vi "GetCreditTransactions.vi"(8 "error in (no error)":errorcluster, 9 "Month":T1, 10 "YYYY":i32, 11 "Account History in":refnum<class "Account History.lvclass">) -> (0 "error out":errorcluster, 2 "Credit Transactions.lvclass":refnum<class "Credit Transactions.lvclass">, 3 "Account History out":refnum<class "Account History.lvclass">)   [LabVIEW 2018, in "Account History.lvclass"]
uses:
  Account History.lvclass
  Credit Statement/Credit Transactions.lvclass
  C:/GitRepos/Filthy-Lucre-Budgetizer/source/support/classes/Statement/TransactionList.lvclass
  Month.ctl
  Credit Record/Credit Transaction.lvclass
  C:/GitRepos/Filthy-Lucre-Budgetizer/source/support/classes/Transaction/Transaction.lvclass
  Statement/TransactionList.lvclass
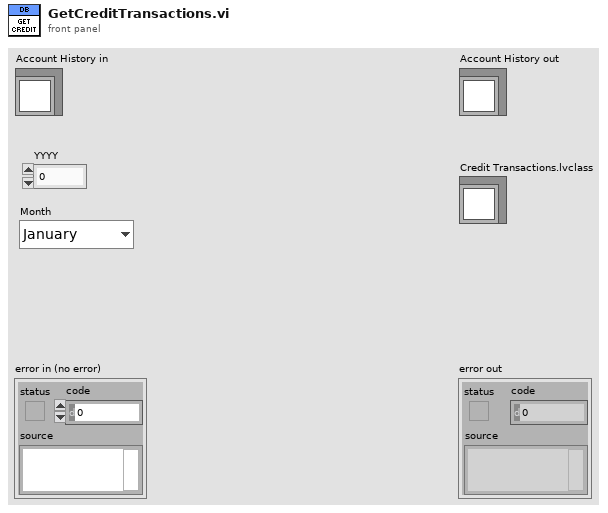
[diagram p1: front panel]
types:
  T1 = typedef "Account History.lvclass/Month.ctl" = enum16{"January", "February", "March", "April", "May", "June", "July", "August", "September", "October", "November", "December"}
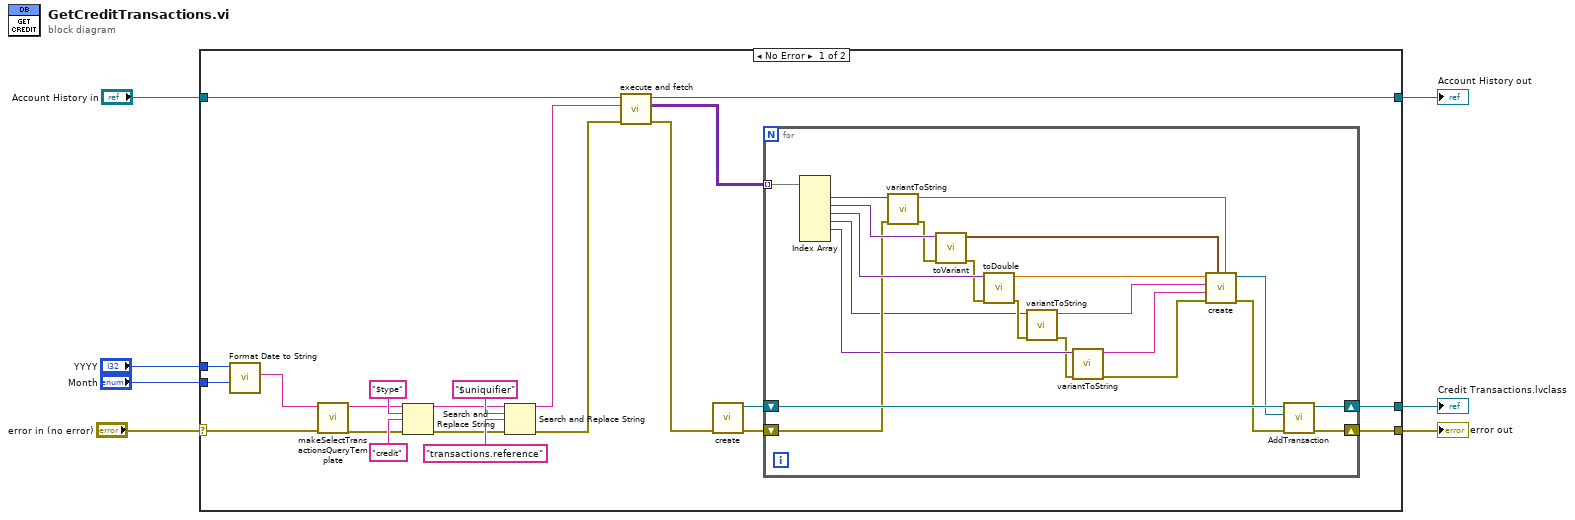
[diagram p0: block diagram]
diagram:
  n1 = case shown="No Error" "error in (no error)" {
    selector: "error in (no error)" -> [w25 w53]
    tunnel: [w13 w53] -> w1
    tunnel: [w26 w52] -> w6
    tunnel: "Account History in" -> [w29 w52]
    tunnel: [w12 _] -> w2
    tunnel: "YYYY" -> [w28 _]
    tunnel: "Month" -> [w27 _]
    frame No Error {
      n2 = call "Format Date to String.vi"("Month"=w27, "YYYY"=w28) -> ("Year-Mo"=w24:string)  [unwired: 9 in]
      n3 = call "makeSelectTransactionsQueryTemplate.vi"("error in (no error)"=w25, "date"=w24) -> ("error out"=w20:errorcluster, "result string"=w21:string)  [unwired: 8 in]
      n4 = Search and Replace String(input string=w21, search string="$type", replace string="credit", error in=w20) -> (result string=w17:string, error out=w16:errorcluster)  [unwired: 4 in, 2 out]
      n5 = Search and Replace String(input string=w17, search string="$uniquifier", replace string="transactions.reference", error in=w16) -> (result string=w14:string, error out=w15:errorcluster)  [unwired: 4 in, 2 out]
      n6 = call "execute and fetch.vi"("error in (no error)"=w15, "SQL query"=w14, "Database in"=w29) -> ("error out"=w9:errorcluster, "recordset data"=w11:variant[][], "Database out"=w26:refnum<class "Account History.lvclass">)  [unwired: 5 in, 1 out]
      n7 = call "create.vi"("error in (no error)"=w9) -> ("error out"=w8:errorcluster, "Credit Transactions out"=w10:refnum<class "Credit Transactions.lvclass">)  [unwired: 9 in]
      n8 = for {
        shift-right: [w50] -> w12
        shift-left: w10 -> [w51]
        shift-right: [w49] -> w13
        shift-left: w8 -> [w37]
        tunnel: w11 -> [w46] mode=indexing
        n9 = Index Array(array=w46) -> (element #1=w45:variant, element #2=w43:variant, element #3=w41:variant, element #4=w33:variant, element #5=w32:variant)  [unwired: 6 in, 1 out]
        n10 = call "variantToString.vi"("error in (no error)"=w37, "Variant"=w45) -> ("error out"=w36:errorcluster, "String"=w44:string)  [unwired: 8 in]
        n11 = call "toVariant.vi"("error in (no error)"=w36, "Variant"=w43) -> ("error out"=w35:errorcluster, "time stamp"=w42:timestamp)  [unwired: 8 in]
        n12 = call "toDouble.vi"("error in (no error)"=w35, "Value"=w41) -> ("error out"=w34:errorcluster, "type"=w40:dbl)  [unwired: 8 in]
        n13 = call "variantToString.vi"("error in (no error)"=w34, "Variant"=w33) -> ("error out"=w31:errorcluster, "String"=w39:string)  [unwired: 8 in]
        n14 = call "variantToString.vi"("error in (no error)"=w31, "Variant"=w32) -> ("error out"=w30:errorcluster, "String"=w38:string)  [unwired: 8 in]
        n15 = call "create.vi"("Reference"=w44, "Date"=w42, "error in (no error)"=w30, "Category"=w38, "Description"=w39, "Amount"=w40) -> ("error out"=w47:errorcluster, "Credit Transaction out"=w48:refnum<class "Credit Transaction.lvclass">)  [unwired: 4 in]
        n16 = call "AddTransaction.vi"("error in (no error)"=w47, "Transaction.lvclass"=w48, "TransactionList in"=w51) -> ("error out"=w49:errorcluster, "TransactionList out"=w50:refnum<class "Credit Transactions.lvclass">)  [unwired: 7 in]
      }
    }
    frame Error {
    }
  }
  "error out" <- w1
  "Account History out" <- w6
  "Credit Transactions.lvclass" <- w2
